vi "Number to Four Bytes.vi"(9 "Fractional Precision (3)":sgl=3.0 format="%#_0p", 10 "Input Value (0)":dbl) -> (0 "Byte 4":i32, 1 "Byte 3":i32, 2 "Byte 2":i32, 3 "Byte 1":i32)   [LabVIEW 2019, in "BK Precision 178XB Series.lvlib"]
doc: "This SubVI takes the <b>Input Value</b> and manipulates the data representation into a fractional value based on <b>Fractional Precision</b>. It then converts the value into four bytes in hexadecimal, then represented in decimal format at the output (Byte 1, Byte2, Byte 3, Byte 4).\n\nThis SubVI is used to convert set values for voltage, current, power, and resistance. The <b>Fractional Precision</b> is used to set the numerical representation used to convert and configure into command frame. For example, 3 is used to convert the input so that 1 represents 1 mV for voltage setup. Likewise, 4 is used to convert current so that 1 represents 0.1 mA in current setup. Refer to user manual for more details."
uses:
  BK Precision 178XB Series.lvlib
panel:
  # "(c) 2009 B&K PRECISION CORPORATION.  ALL RIGHTS RESERVED."
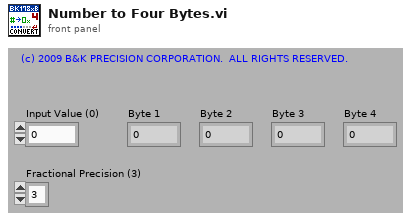
[diagram p1: front panel]
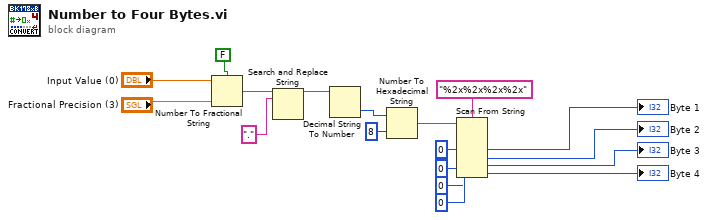
[diagram p0: block diagram]
diagram:
  n1 = Number To Fractional String(use system decimal point (T)=FALSE, number="Input Value (0)", precision (6)="Fractional Precision (3)") -> (F-format string=w4:string)  [unwired: 1 in]
  n2 = Search and Replace String(input string=w4, search string=".") -> (result string=w6:string)  [unwired: 6 in, 3 out]
  n3 = Decimal String To Number(string=w6) -> (number=w7:i32)  [unwired: 2 in, 1 out]
  n4 = Number To Hexadecimal String(1:i16 8 ("width (-)"), 2:w7) -> (0:w9:string)
  n5 = Scan From String(format string="%2x%2x%2x%2x", input string=w9, default 1=0 ("default value 1"), default 2=0 ("default value 2"), default 3=0 ("default value 3"), default 4=0 ("default value 4")) -> (output 1=→"Byte 1":i32, output 2=→"Byte 2":i32, output 3=→"Byte 3":i32, output 4=→"Byte 4":i32)  [unwired: 2 in, 3 out]
